vi "oa_Build Spectral Info for Order Magnitude and Phase (1 Channel).vi"(0 "resampled channel info":T8={"channel name"="", "description"="", " channel info"={"sensor sensitivity"=1000.0, "engineering units"=1, "dB reference"=1.0, "custom label"="EU", "weighting filter"=0, "pregain"=0.0}} {"channel info"."pregain" format="%.2f"; "channel info"."weighting filter" items=["Linear", "A-weighting", "B-weighting", "C-weighting", "ITU-R 468-4", "Dolby", "CCITT", "C-message", "Wb", "Wc", "Wd", "We", "Wf", "Wh", "Wj", "Wk", "Wm", "AES17 20 kHz lowpass", "AES17 40 kHz lowpass", "AES17 20 kHz highpass", "AES17 40 kHz highpass"]; "channel info"."dB reference" format="%^.1e"; "channel info"."engineering units" items=["custom..."=0, "V"=1, "A"=21, "C"=30, "pC"=31, "s"=32, "-"=29, "Pa"=2, "N"=20, "g"=3, "m/s^2"=4, "m/s"=5, "m"=6, "mm/s"=12, "mm"=13, "micron/s"=14, "micron"=15, "in/s^2"=7, "in/s"=8, "in"=9, "mil/s"=10, "mil"=11, "rad/s^2"=16, "rad/s"=17, "rad"=18, "deg/s^2"=26, "deg/s"=27, "deg"=28, "RPM"=22, "cycle/s^2"=23, "Hz"=24, "cycle"=25, "strain"=19]; "channel info"."sensor sensitivity" format="%#_5f"}, 1 "reset? (T)":bool=TRUE, 5 "X axis selection":u16(ring)=2 items=["Time", "Revolution", "RPM"], 7 "unit label":string, 9 "orders to compute":dbl[](array[numeric]) format="%.2f", 11 "error in (no error)":errorcluster, 12 "view":T1={"dB on? (T)"=FALSE, "unwrap phase? (T)"=TRUE, "unit in degree? (T)"=TRUE}) -> (4 "spectrum info":T2={"channel name"="", "description"="", "x-axis units"=0, "spectral info"={"spectrum type"=enum."Power [Magnitude^2]", "linear/dB"=enum."linear", "window"=0, "window size"=0, "FFT size"=0}, "engineering units"=1, "custom label"="", "dB reference [EU]"=0.0, "peak units"=enum."rms", "weighting filter"=0, "spectral density?"=FALSE, "unit label"="", "spectrum skewed?"=FALSE, "complimentary spectrum units"=enum."none"} {"x-axis units" items=["Time (s)"=0, "Frequency-CB (Hz)"=1, "Frequency-CPB (Hz)"=1248, "Frequency-Arbitrary (Hz)"=2357, "Quefrency (s)"=2, "Revolutions (rev)"=3, "Order"=4, "Speed (RPM)"=11, "Speed (rad/s)"=21, "Index"=65535]; "weighting filter" items=["Linear", "A-weighting", "B-weighting", "C-weighting", "ITU-R 468-4", "Dolby", "CCITT", "C-message", "Wb", "Wc", "Wd", "We", "Wf", "Wh", "Wj", "Wk", "Wm", "AES17 20 kHz lowpass", "AES17 40 kHz lowpass", "AES17 20 kHz highpass", "AES17 40 kHz highpass"]; "dB reference [EU]" format="%.2f"; "engineering units" items=["custom..."=0, "V"=1, "A"=21, "C"=30, "pC"=31, "s"=32, "-"=29, "Pa"=2, "N"=20, "g"=3, "m/s^2"=4, "m/s"=5, "m"=6, "mm/s"=12, "mm"=13, "micron/s"=14, "micron"=15, "in/s^2"=7, "in/s"=8, "in"=9, "mil/s"=10, "mil"=11, "rad/s^2"=16, "rad/s"=17, "rad"=18, "deg/s^2"=26, "deg/s"=27, "deg"=28, "RPM"=22, "cycle/s^2"=23, "Hz"=24, "cycle"=25, "strain"=19]; "spectral info"."window" items=["None "=0, "Hanning"=1, "Hamming"=2, "Blackman-Harris"=3, "Exact Blackman"=4, "Blackman"=5, "Flat Top"=6, "4 Term B-Harris "=7, "7 Term B-Harris"=8, "Low Sidelobe"=9, "Force - Exponential"=10, "Gaussian"=62]}, 15 "error out":errorcluster)   [LabVIEW 2017, in "SoundVib_Resampling.lvlib"]
uses:
  <vilib>/addons/Sound and Vibration/Order Analysis/Resample Order Tracking/SoundVib_Resampling.lvlib
  <vilib>/addons/_NISVFA/_Shared subVIs/Controls/svc_Resampled Channel Info.ctl
  <vilib>/addons/_NISVFA/_Shared subVIs/Controls/svc_Channel Info.ctl
  <vilib>/addons/_NISVFA/_Shared subVIs/Controls/svc_Engineering Units Text Ring.ctl
  <vilib>/addons/_NISVFA/_Shared subVIs/Controls/svc_Weighting Filter Text Ring.ctl
  <vilib>/addons/_NISVFA/_Shared subVIs/Controls/svc_Spectrum Info.ctl
  <vilib>/addons/_NISVFA/_Shared subVIs/Controls/svc_X-Axis Units.ctl
  <vilib>/addons/_NISVFA/_Shared subVIs/Controls/svc_Spectrum Type.ctl
  <vilib>/addons/_NISVFA/_Shared subVIs/Controls/svc_Complimentary Spectrum Units.ctl
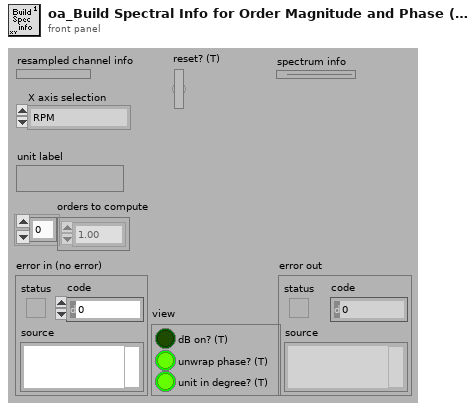
[diagram p1: front panel]
types:
  T1 = cluster{"dB on? (T)":bool, "unwrap phase? (T)":bool, "unit in degree? (T)":bool}
  T2 = typedef "svc_Spectrum Info.ctl" = cluster{"channel name":string, "description":string, "x-axis units":T3, "spectral info":cluster{"spectrum type":T4, "linear/dB":enum16{"linear", "dB"}, "window":u16, "window size":i32, "FFT size":i32}, "engineering units":T5, "custom label":string, "dB reference [EU]":dbl, "peak units":enum16{"rms", "peak", "peak-peak"}, "weighting filter":T6, "spectral density?":bool, "unit label":string, "spectrum skewed?":bool, "complimentary spectrum units":T7}
  T3 = typedef "svc_X-Axis Units.ctl" = u16
  T4 = typedef "svc_Spectrum Type.ctl" = enum16{"FFT Spectrum [complex]", "Amplitude [Magnitude]", "Power [Magnitude^2]", "Cross Spectrum [complex]", "Frequency Response [Complex]"}
  T5 = typedef "svc_Engineering Units Text Ring.ctl" = u16
  T6 = typedef "svc_Weighting Filter Text Ring.ctl" = u16
  T7 = typedef "svc_Complimentary Spectrum Units.ctl" = enum16{"none", "radians", "degrees", "cycles", "imaginary"}
  T8 = typedef "svc_Resampled Channel Info.ctl" = cluster{"channel name":string, "description":string, " channel info":T9}
  T9 = typedef "svc_Channel Info.ctl" = cluster{"sensor sensitivity":dbl, "engineering units":T5, "dB reference":dbl, "custom label":string, "weighting filter":T6, "pregain":dbl}
  T10 = cluster{"spectrum type":T4, "linear/dB":enum16{"linear", "dB"}, "window":u16, "window size":i32, "FFT size":i32}
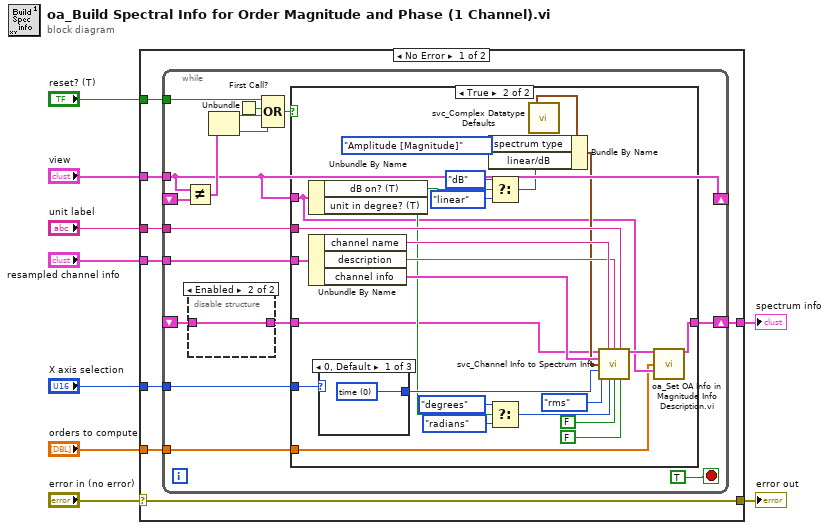
[diagram p0: block diagram]
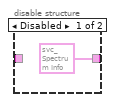
[diagram p2: hidden frame]
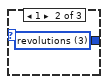
[diagram p4: hidden frame]
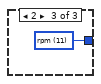
[diagram p5: hidden frame]
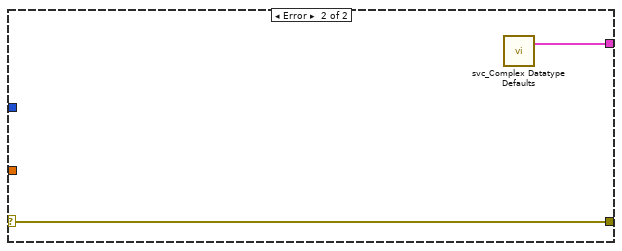
[diagram p6: hidden frame]
diagram:
  n1 = case shown="No Error" "error in (no error)" {
    selector: "error in (no error)" -> [w16 w67]
    tunnel: [w16 w67] -> w8
    tunnel: [w14 w66] -> w7
    tunnel: "resampled channel info" -> [w17 _]
    tunnel: "unit label" -> [w13 _]
    tunnel: "X axis selection" -> [w15 _]
    tunnel: "view" -> [w12 _]
    tunnel: "reset? (T)" -> [w11 _]
    tunnel: "orders to compute" -> [w10 _]
    frame No Error {
      n2 = while {
        tunnel: w17 -> [w33]
        tunnel: w15 -> [w32]
        tunnel: w13 -> [w30]
        tunnel: w12 -> [w22]
        tunnel: w11 -> [w29]
        shift-right: [w22] -> _
        shift-left: _ -> [w21]
        shift-right: [w31] -> w14
        shift-left: _ -> [w18]
        tunnel: w10 -> [w20]
        stop <- TRUE stop-if-true
        n3 = Not Equal?(x=w22, y=w21) -> (x != y?=w27:T1)
        n4 = disable-structure shown="Enabled" {
          disable-tunnel: [T2 {"channel name"="", "description"="", "x-axis units"=0, "spectral info"={"spectrum type"=enum."Power [Magnitude^2]", "linear/dB"=enum."linear", "window"=0, "window size"=0, "FFT size"=0}, "engineering units"=1, "custom label"="", "dB reference [EU]"=0.0, "peak units"=enum."rms", "weighting filter"=0, "spectral density?"=FALSE, "unit label"="", "spectrum skewed?"=FALSE, "complimentary spectrum units"=enum."none"} ("magnitude info out") w35] -> w19
          disable-tunnel: w18 -> [_ w35]
          frame Disabled {
          }
          frame Enabled {
          }
        }
        n5 = Unbundle(w27) -> ("dB on? (T)"=w26:bool, "unit in degree? (T)"=w25:bool)  [unwired: 1 out]
        n6 = First Call?() -> (First Call?: T/F=w28:bool)
        n7 = Compound Arithmetic op=OR(w29, w28, w26, w25) -> (w24:bool)
        n8 = case shown="True" w24 {
          tunnel: w33 -> [_ w62]
          tunnel: w32 -> [_ w61]
          tunnel: [w36 w39] -> w31
          tunnel: w30 -> [_ w58]
          tunnel: w22 -> [_ w38]
          tunnel: w19 -> [w36 w41]
          tunnel: w20 -> [_ w37]
          frame False {
          }
          frame True {
            n9 = Unbundle By Name(w38) -> ("dB on? (T)"=w46:bool, "unit in degree? (T)"=w44:bool)
            n10 = Unbundle By Name(w62) -> ("channel name"=w60:string, "description"=w59:string, "channel info"=w55:T9)
            n11 = case shown="0, Default" w61 {
              tunnel: [w63 w64 w65] -> w53
              frame 0, Default {
                w63 = u16 0 items=["time"=0, "frequency"=1, "quefrency"=2, "revolutions"=3, "order"=4, "rpm"=11] ("x-axis units")
              }
              frame 1 {
                w64 = u16 3 items=["time"=0, "frequency"=1, "quefrency"=2, "revolutions"=3, "order"=4, "rpm"=11] ("x-axis units")
              }
              frame 2 {
                w65 = u16 11 items=["time"=0, "frequency"=1, "quefrency"=2, "revolutions"=3, "order"=4, "rpm"=11] ("x-axis units")
              }
            }
            n12 = Select(t=enum16{"linear", "dB"}."dB" ("spectral info.linear/dB"), s=w46, f=enum16{"linear", "dB"}."linear" ("spectral info.linear/dB")) -> (s? t:f=w47:enum16{"linear", "dB"})
            n13 = Select(t=svc_Complimentary_Spectrum_Units."degrees" ("complimentary spectrum units"), s=w44, f=svc_Complimentary_Spectrum_Units."radians" ("complimentary spectrum units")) -> (s? t:f=w43:T7)
            n14 = call <vilib>:"svc_Complex Datatype Defaults.vi"() -> ("spectral info"=w50:T10)  [unwired: 11 in, 8 out]
            n15 = Bundle By Name(cluster=w50, "spectrum type"=svc_Spectrum_Type."Amplitude [Magnitude]", "linear/dB"=w47) -> (w49:T10)
            n16 = call <vilib>:"svc_Channel Info to Spectrum Info.vi"("spectrum info in"=w41, "channel name"=w60, "description"=w59, "unit label"=w58, "channel info"=w55, "spectral info"=w49, "x-axis units"=w53, "peak units"=enum16{"rms", "peak", "peak-peak"}."rms", "complimentary spectrum units"=w43, "spectral density?"=FALSE, "spectrum skewed?"=FALSE) -> ("spectrum info out"=w40:T2)  [unwired: 4 in]
            n17 = call <vilib>:"oa_Set OA Info in Magnitude Info Description.vi.vi"("magnitude info"=w40, "orders to compute"=w37, "view"=w38) -> ("magnitude info out"=w39:T2)  [unwired: 11 in, 1 out]
          }
        }
      }
    }
    frame Error {
      n18 = call <vilib>:"svc_Complex Datatype Defaults.vi"() -> ("dead spectrum info"=w66:T2)  [unwired: 11 in, 8 out]
    }
  }
  "error out" <- w8
  "spectrum info" <- w7
